vi "Get Strings from Ref.vi"(8 "error in (no error)":errorcluster, 9 "Label Prefix":string, 10 "GObj Refnum in":refnum<vi>, 11 "GraphChart in":refnum<class "GraphChart.lvclass">) -> (0 "error out":errorcluster, 1 "Valid?":bool, 2 "GObj Refnum out":refnum<vi>, 3 "GraphChart out":refnum<class "GraphChart.lvclass">, 4 "GObj Name":string)   [LabVIEW 2013, in "SET Project Data.lvlib" / "GraphChart.lvclass"]
uses:
  GraphChart.lvclass
  Control/Control.lvclass
  GObject/GObject.lvclass/GObject.ctl
  GObject/Write UID.vi
  SET Project Data.lvlib
  GObject/GObject.lvclass
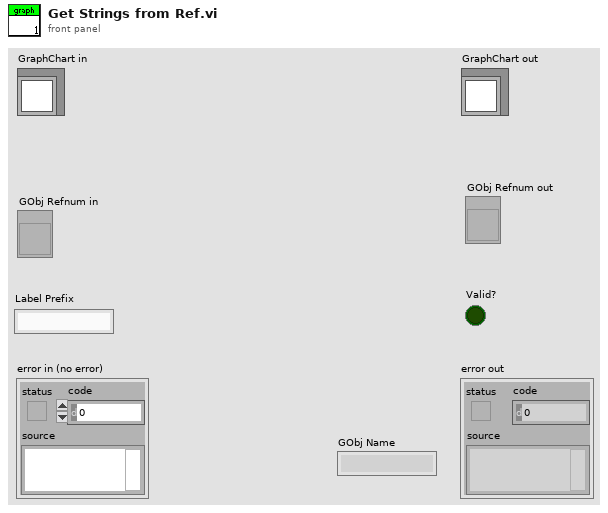
[diagram p1: front panel]
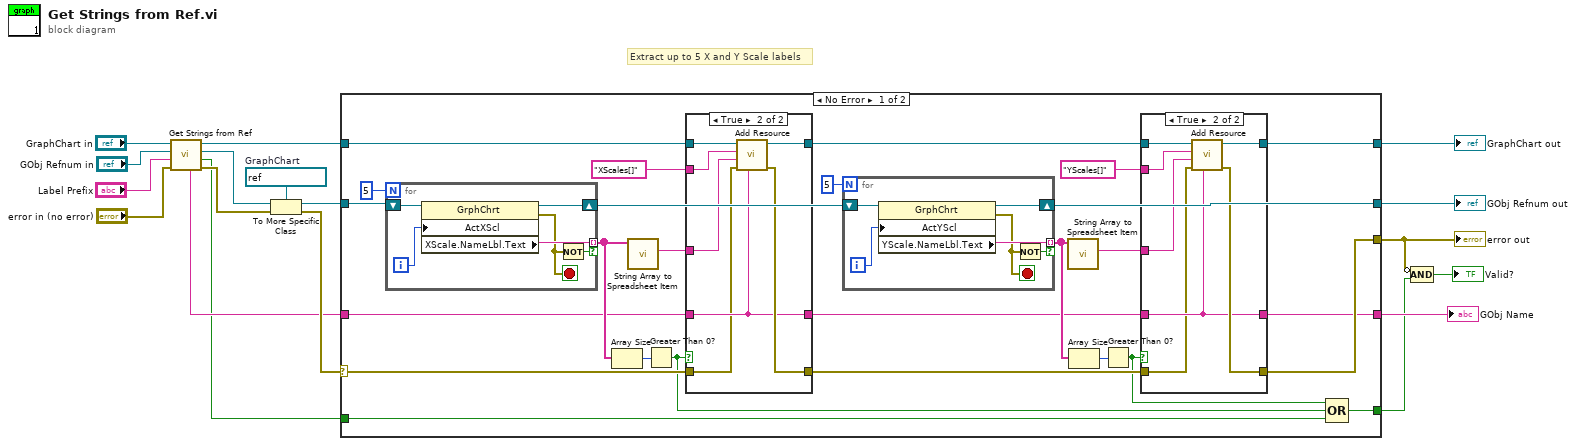
[diagram p0: block diagram]
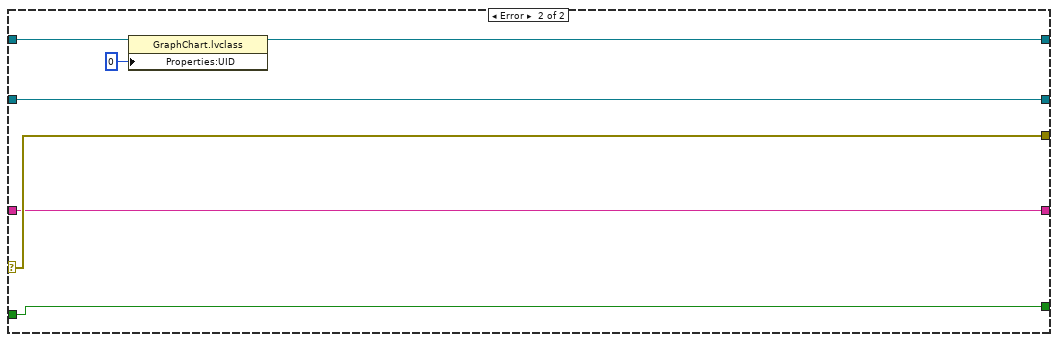
[diagram p4: hidden frame]
diagram:
  w15 = refnum<vi> refnum  # GraphChart
  # "Extract up to 5 X and Y Scale labels"
  n1 = call-parent "Get Strings from Ref.vi"("error in (no error)"="error in (no error)", "Label Prefix"="Label Prefix", "GObj Refnum in"="GObj Refnum in", "Control in"="GraphChart in") -> ("error out"=w14:errorcluster, "Valid?"=w3:bool, "GObj Refnum out"=w13:refnum<vi>, "Control out"=w18:refnum<class "GraphChart.lvclass">, "GObj Name"=w4:string)  [unwired: 3 in]
  n2 = To More Specific Class(target class=w15, reference=w13, error in=w14) -> (specific class reference=w16:refnum<vi>, error out=w17:errorcluster)
  n3 = case shown="No Error" w17 {
    selector: w17 -> [w31 w82]
    tunnel: w16 -> [w44 w83]
    tunnel: w18 -> [w35 w81]
    tunnel: [w30 w79] -> w11
    tunnel: [w24 w82] -> w7
    tunnel: [w41 w83] -> w5
    tunnel: w4 -> [w32 w78]
    tunnel: w3 -> [w20 w77]
    tunnel: [w23 w78] -> w2
    tunnel: [w19 w77] -> w1
    frame No Error {
      n4 = for {
        N: 5 -> [_]
        shift-right: [w75] -> w42
        shift-left: w44 -> [w76]
        tunnel: [w73] -> w39 mode=indexing if=w72
        i -> [w74]
        stop <- w71 stop-if-true
        n5 = property class="GrphChrt"(reference=w76, "ActXScl"=w74) -> (reference out=w75:refnum<vi>, error out=w71:errorcluster, "XScale.NameLbl.Text"=w73:string)  [unwired: 1 in]
        n6 = Not(x=w71) -> (.not. x?=w72:bool)
      }
      n7 = Array Size(array=w39) -> (size(s)=w40:i32)
      n8 = call "String Array to Spreadsheet Item.vi"("Strings [] (ASCII)"=w39) -> ("Spreadsheet Item (ASCII)"=w33:string)  [unwired: 10 in]
      n9 = Greater Than 0?(x=w40) -> (x > 0?=w21:bool)
      n10 = case shown="True" w21 {
        tunnel: w35 -> [w57 w64]
        tunnel: [w57 w63] -> w29
        tunnel: w32 -> [w56 w59]
        tunnel: w33 -> [_ w62]
        tunnel: "XScales[]" -> [_ w61]
        tunnel: [w55 w60] -> w25
        tunnel: [w56 w59] -> w26
        tunnel: w31 -> [w55 w58]
        frame False {
        }
        frame True {
          n11 = call "Add Resource.vi"("TagPrefix"=w59, "error in (no error)"=w58, "ItemText"=w62, "ItemName"=w61, "GObject in"=w64) -> ("error out"=w60:errorcluster, "GObject out"=w63:refnum<class "GraphChart.lvclass">)  [unwired: 5 in]
        }
      }
      n12 = for {
        N: 5 -> [_]
        shift-right: [w69] -> w41
        shift-left: w42 -> [w70]
        tunnel: [w67] -> w37 mode=indexing if=w66
        i -> [w68]
        stop <- w65 stop-if-true
        n13 = property class="GrphChrt"(reference=w70, "ActYScl"=w68) -> (reference out=w69:refnum<vi>, error out=w65:errorcluster, "YScale.NameLbl.Text"=w67:string)  [unwired: 1 in]
        n14 = Not(x=w65) -> (.not. x?=w66:bool)
      }
      n15 = call "String Array to Spreadsheet Item.vi"("Strings [] (ASCII)"=w37) -> ("Spreadsheet Item (ASCII)"=w27:string)  [unwired: 10 in]
      n16 = Array Size(array=w37) -> (size(s)=w38:i32)
      n17 = Greater Than 0?(x=w38) -> (x > 0?=w22:bool)
      n18 = case shown="True" w22 {
        tunnel: w29 -> [w47 w54]
        tunnel: [w47 w53] -> w30
        tunnel: w26 -> [w46 w49]
        tunnel: w27 -> [_ w52]
        tunnel: "YScales[]" -> [_ w51]
        tunnel: [w45 w50] -> w24
        tunnel: [w46 w49] -> w23
        tunnel: w25 -> [w45 w48]
        frame False {
        }
        frame True {
          n19 = call "Add Resource.vi"("TagPrefix"=w49, "error in (no error)"=w48, "ItemText"=w52, "ItemName"=w51, "GObject in"=w54) -> ("error out"=w50:errorcluster, "GObject out"=w53:refnum<class "GraphChart.lvclass">)  [unwired: 5 in]
        }
      }
      n20 = Compound Arithmetic op=OR(w22, w21, w20) -> (w19:bool)
    }
    frame Error {
      n21 = property class="GraphChart.lvclass"(reference=w81, "Properties:UID"=0 ("UID")) -> (reference out=w79:refnum<class "GraphChart.lvclass">)  [unwired: 1 in, 1 out]
    }
  }
  "error out" <- w7
  "GraphChart out" <- w11
  "GObj Refnum out" <- w5
  "GObj Name" <- w2
  n22 = Compound Arithmetic op=AND(invert w7, w1) -> (→"Valid?":bool)
